vi "Line Linear Fit.vi"(8 "error in":errorcluster, 9 "Keys":refnum<class "1D Array u32.lvclass">, 10 "Y":refnum<class "1D Array f32.lvclass">, 11 "X":refnum<class "1D Array f32.lvclass">) -> (0 "error out":errorcluster, 1 "Keys":refnum<class "1D Array u32.lvclass">, 2 "Offset":refnum<class "1D Array f32.lvclass">, 3 "Slope":refnum<class "1D Array f32.lvclass">)   [LabVIEW 2024, in "G2CPU Line Profile.lvlib"]
uses:
  G2CPU Line Profile.lvlib
  <vilib>/Natan Biesmans/G2CPU GPU and CPU HPC Toolkit/G2CPU Libraries/Arrays/1DArray/f32/1D Array f32.lvclass
  C:/Program Files/National Instruments/LabVIEW 2025/vi.lib/Natan Biesmans/G2CPU GPU and CPU HPC Toolkit/G2CPU Libraries/Arrays/Array/Array Prototype.lvclass
  C:/Program Files/National Instruments/LabVIEW 2025/vi.lib/Natan Biesmans/G2CPU GPU and CPU HPC Toolkit/G2CPU Libraries/Arrays/1DArray/1D Array Prototype.lvclass
  <vilib>/Natan Biesmans/G2CPU GPU and CPU HPC Toolkit/G2CPU Libraries/Arrays/1DArray/u32/1D Array u32.lvclass
  168ab924-3f3a-4db2-9cdf-e3d1f64b3aa0.vi
  0e2f45cd-41b9-45c1-a9b9-d013222e4af8.vi
  1f0995f6-d0b0-43f5-a6c2-40305d76432c.vi
  3dc9b0e7-5c3c-4335-af04-05c96a1d9579.vi
  eb82d686-69ce-41bb-8ade-32c9401aa96d.vi
  546f2740-fcf4-4d92-a73d-2c7a874bd7f8.vi
  a3d83607-c738-4256-a254-dc9f631af114.vi
  ee062472-8682-463b-83ff-a41c4e45bcd6.vi
  10035bee-21f0-4aab-9f26-4981b32c8c4e.vi
  73cb6350-5534-4d8a-b705-d1efc928d9b2.vi
  14413830-6ba5-421c-b5be-a333aee7ddc9.vi
  661186f9-425e-4888-8acc-81e64f3364c9.vi
  700b6014-a647-433f-a561-5befaa5067fc.vi
  6550b275-f30d-4b92-a02f-5e7bb5c687a5.vi
  820307c5-4fb2-499f-9659-8297cac63ad2.vi
  c3e4c011-86fb-4641-86fe-1625446fe100.vi
  84420d7e-1cd2-4cf3-975b-0a4a3f4d0c7e.vi
  168ab924-3f3a-4db2-9cdf-e3d1f64b3aa0.vi/6e6c067d-5978-424b-80f1-88c3a0ffd5ec.vi
  168ab924-3f3a-4db2-9cdf-e3d1f64b3aa0.vi/102d6add-a795-4112-b477-17e7a72fc443.vi
  168ab924-3f3a-4db2-9cdf-e3d1f64b3aa0.vi/cd277467-b234-4cce-8fd2-a3bd8d6792e1.vi
  0e2f45cd-41b9-45c1-a9b9-d013222e4af8.vi/6197f869-f6d4-49b3-9b2c-cc979b422c2e.vi
  0e2f45cd-41b9-45c1-a9b9-d013222e4af8.vi/a7e86dbb-b4c0-485c-89c5-522e60ee265c.vi
  1f0995f6-d0b0-43f5-a6c2-40305d76432c.vi/d0fc544b-4239-492d-8a0f-f99369e9c7ae.vi
  1f0995f6-d0b0-43f5-a6c2-40305d76432c.vi/3d9e75e3-2a93-4e4c-a851-83639de319bb.vi
  3dc9b0e7-5c3c-4335-af04-05c96a1d9579.vi/c9dded55-ca8d-4e9c-82fa-de3705eb1997.vi
  3dc9b0e7-5c3c-4335-af04-05c96a1d9579.vi/77657c34-d6a5-4eb3-ad2b-a32f9da8910d.vi
  eb82d686-69ce-41bb-8ade-32c9401aa96d.vi/6197f869-f6d4-49b3-9b2c-cc979b422c2e.vi
  eb82d686-69ce-41bb-8ade-32c9401aa96d.vi/a7e86dbb-b4c0-485c-89c5-522e60ee265c.vi
  546f2740-fcf4-4d92-a73d-2c7a874bd7f8.vi/c9dded55-ca8d-4e9c-82fa-de3705eb1997.vi
  546f2740-fcf4-4d92-a73d-2c7a874bd7f8.vi/77657c34-d6a5-4eb3-ad2b-a32f9da8910d.vi
  a3d83607-c738-4256-a254-dc9f631af114.vi/c9dded55-ca8d-4e9c-82fa-de3705eb1997.vi
  a3d83607-c738-4256-a254-dc9f631af114.vi/77657c34-d6a5-4eb3-ad2b-a32f9da8910d.vi
  ee062472-8682-463b-83ff-a41c4e45bcd6.vi/6197f869-f6d4-49b3-9b2c-cc979b422c2e.vi
  ee062472-8682-463b-83ff-a41c4e45bcd6.vi/a7e86dbb-b4c0-485c-89c5-522e60ee265c.vi
  10035bee-21f0-4aab-9f26-4981b32c8c4e.vi/c9dded55-ca8d-4e9c-82fa-de3705eb1997.vi
  10035bee-21f0-4aab-9f26-4981b32c8c4e.vi/77657c34-d6a5-4eb3-ad2b-a32f9da8910d.vi
  73cb6350-5534-4d8a-b705-d1efc928d9b2.vi/6197f869-f6d4-49b3-9b2c-cc979b422c2e.vi
  73cb6350-5534-4d8a-b705-d1efc928d9b2.vi/a7e86dbb-b4c0-485c-89c5-522e60ee265c.vi
  14413830-6ba5-421c-b5be-a333aee7ddc9.vi/1bf6e03b-eb75-45f6-9764-49dc38a3a024.vi
  14413830-6ba5-421c-b5be-a333aee7ddc9.vi/2da4419f-02df-47a7-be00-1b7e0871fa33.vi
  661186f9-425e-4888-8acc-81e64f3364c9.vi/d0fc544b-4239-492d-8a0f-f99369e9c7ae.vi
  661186f9-425e-4888-8acc-81e64f3364c9.vi/3d9e75e3-2a93-4e4c-a851-83639de319bb.vi
  700b6014-a647-433f-a561-5befaa5067fc.vi/1bf6e03b-eb75-45f6-9764-49dc38a3a024.vi
  700b6014-a647-433f-a561-5befaa5067fc.vi/2da4419f-02df-47a7-be00-1b7e0871fa33.vi
  6550b275-f30d-4b92-a02f-5e7bb5c687a5.vi/46771f49-eb1d-473b-8e81-f516cef50a4e.vi
  6550b275-f30d-4b92-a02f-5e7bb5c687a5.vi/dc76f8e4-64fa-456a-8549-7a4b6936c4c9.vi
  6550b275-f30d-4b92-a02f-5e7bb5c687a5.vi/7e60ddfb-e748-4c0c-85da-e395a1b7978d.vi
  6550b275-f30d-4b92-a02f-5e7bb5c687a5.vi/d2eceff7-f641-4ce4-acfa-e9e293a3c877.vi
  6550b275-f30d-4b92-a02f-5e7bb5c687a5.vi/b737122b-4036-448b-abd3-e2701355e828.vi
  820307c5-4fb2-499f-9659-8297cac63ad2.vi/6197f869-f6d4-49b3-9b2c-cc979b422c2e.vi
  820307c5-4fb2-499f-9659-8297cac63ad2.vi/a7e86dbb-b4c0-485c-89c5-522e60ee265c.vi
  c3e4c011-86fb-4641-86fe-1625446fe100.vi/1bf6e03b-eb75-45f6-9764-49dc38a3a024.vi
  c3e4c011-86fb-4641-86fe-1625446fe100.vi/2da4419f-02df-47a7-be00-1b7e0871fa33.vi
  84420d7e-1cd2-4cf3-975b-0a4a3f4d0c7e.vi/46771f49-eb1d-473b-8e81-f516cef50a4e.vi
  84420d7e-1cd2-4cf3-975b-0a4a3f4d0c7e.vi/dc76f8e4-64fa-456a-8549-7a4b6936c4c9.vi
  84420d7e-1cd2-4cf3-975b-0a4a3f4d0c7e.vi/7e60ddfb-e748-4c0c-85da-e395a1b7978d.vi
  84420d7e-1cd2-4cf3-975b-0a4a3f4d0c7e.vi/d2eceff7-f641-4ce4-acfa-e9e293a3c877.vi
  84420d7e-1cd2-4cf3-975b-0a4a3f4d0c7e.vi/b737122b-4036-448b-abd3-e2701355e828.vi
  0e2f45cd-41b9-45c1-a9b9-d013222e4af8.vi/6197f869-f6d4-49b3-9b2c-cc979b422c2e.vi/3e802c67-fb96-46a3-ae13-4994a8508b4f.vi
  0e2f45cd-41b9-45c1-a9b9-d013222e4af8.vi/6197f869-f6d4-49b3-9b2c-cc979b422c2e.vi/5a50fc67-79e7-4972-80c2-92243cd53dd4.vi
  0e2f45cd-41b9-45c1-a9b9-d013222e4af8.vi/a7e86dbb-b4c0-485c-89c5-522e60ee265c.vi/730f6c57-5c0b-4ee9-b61e-75067b25222b.vi
  0e2f45cd-41b9-45c1-a9b9-d013222e4af8.vi/a7e86dbb-b4c0-485c-89c5-522e60ee265c.vi/096b8799-7810-404e-baca-ba9279cec4bd.vi
  0e2f45cd-41b9-45c1-a9b9-d013222e4af8.vi/a7e86dbb-b4c0-485c-89c5-522e60ee265c.vi/0f1a5a47-bcc5-4796-ac31-8dfcfbc0d7d1.vi
  0e2f45cd-41b9-45c1-a9b9-d013222e4af8.vi/a7e86dbb-b4c0-485c-89c5-522e60ee265c.vi/89f12e17-3330-4b72-ad8f-8dd636660732.vi
  1f0995f6-d0b0-43f5-a6c2-40305d76432c.vi/d0fc544b-4239-492d-8a0f-f99369e9c7ae.vi/3587aa3f-97a0-4074-a424-c31da557ec96.vi
  1f0995f6-d0b0-43f5-a6c2-40305d76432c.vi/d0fc544b-4239-492d-8a0f-f99369e9c7ae.vi/6058dca8-195d-4566-b47b-6d6a1c5af61f.vi
  1f0995f6-d0b0-43f5-a6c2-40305d76432c.vi/3d9e75e3-2a93-4e4c-a851-83639de319bb.vi/730f6c57-5c0b-4ee9-b61e-75067b25222b.vi
  1f0995f6-d0b0-43f5-a6c2-40305d76432c.vi/3d9e75e3-2a93-4e4c-a851-83639de319bb.vi/096b8799-7810-404e-baca-ba9279cec4bd.vi
  1f0995f6-d0b0-43f5-a6c2-40305d76432c.vi/3d9e75e3-2a93-4e4c-a851-83639de319bb.vi/0f1a5a47-bcc5-4796-ac31-8dfcfbc0d7d1.vi
  1f0995f6-d0b0-43f5-a6c2-40305d76432c.vi/3d9e75e3-2a93-4e4c-a851-83639de319bb.vi/89f12e17-3330-4b72-ad8f-8dd636660732.vi
  eb82d686-69ce-41bb-8ade-32c9401aa96d.vi/6197f869-f6d4-49b3-9b2c-cc979b422c2e.vi/3e802c67-fb96-46a3-ae13-4994a8508b4f.vi
  eb82d686-69ce-41bb-8ade-32c9401aa96d.vi/6197f869-f6d4-49b3-9b2c-cc979b422c2e.vi/5a50fc67-79e7-4972-80c2-92243cd53dd4.vi
  eb82d686-69ce-41bb-8ade-32c9401aa96d.vi/a7e86dbb-b4c0-485c-89c5-522e60ee265c.vi/730f6c57-5c0b-4ee9-b61e-75067b25222b.vi
  eb82d686-69ce-41bb-8ade-32c9401aa96d.vi/a7e86dbb-b4c0-485c-89c5-522e60ee265c.vi/096b8799-7810-404e-baca-ba9279cec4bd.vi
  eb82d686-69ce-41bb-8ade-32c9401aa96d.vi/a7e86dbb-b4c0-485c-89c5-522e60ee265c.vi/0f1a5a47-bcc5-4796-ac31-8dfcfbc0d7d1.vi
  eb82d686-69ce-41bb-8ade-32c9401aa96d.vi/a7e86dbb-b4c0-485c-89c5-522e60ee265c.vi/89f12e17-3330-4b72-ad8f-8dd636660732.vi
  ee062472-8682-463b-83ff-a41c4e45bcd6.vi/6197f869-f6d4-49b3-9b2c-cc979b422c2e.vi/3e802c67-fb96-46a3-ae13-4994a8508b4f.vi
  ee062472-8682-463b-83ff-a41c4e45bcd6.vi/6197f869-f6d4-49b3-9b2c-cc979b422c2e.vi/5a50fc67-79e7-4972-80c2-92243cd53dd4.vi
  ee062472-8682-463b-83ff-a41c4e45bcd6.vi/a7e86dbb-b4c0-485c-89c5-522e60ee265c.vi/730f6c57-5c0b-4ee9-b61e-75067b25222b.vi
  ee062472-8682-463b-83ff-a41c4e45bcd6.vi/a7e86dbb-b4c0-485c-89c5-522e60ee265c.vi/096b8799-7810-404e-baca-ba9279cec4bd.vi
  ee062472-8682-463b-83ff-a41c4e45bcd6.vi/a7e86dbb-b4c0-485c-89c5-522e60ee265c.vi/0f1a5a47-bcc5-4796-ac31-8dfcfbc0d7d1.vi
  ee062472-8682-463b-83ff-a41c4e45bcd6.vi/a7e86dbb-b4c0-485c-89c5-522e60ee265c.vi/89f12e17-3330-4b72-ad8f-8dd636660732.vi
  73cb6350-5534-4d8a-b705-d1efc928d9b2.vi/6197f869-f6d4-49b3-9b2c-cc979b422c2e.vi/3e802c67-fb96-46a3-ae13-4994a8508b4f.vi
  73cb6350-5534-4d8a-b705-d1efc928d9b2.vi/6197f869-f6d4-49b3-9b2c-cc979b422c2e.vi/5a50fc67-79e7-4972-80c2-92243cd53dd4.vi
  73cb6350-5534-4d8a-b705-d1efc928d9b2.vi/a7e86dbb-b4c0-485c-89c5-522e60ee265c.vi/730f6c57-5c0b-4ee9-b61e-75067b25222b.vi
  73cb6350-5534-4d8a-b705-d1efc928d9b2.vi/a7e86dbb-b4c0-485c-89c5-522e60ee265c.vi/096b8799-7810-404e-baca-ba9279cec4bd.vi
  73cb6350-5534-4d8a-b705-d1efc928d9b2.vi/a7e86dbb-b4c0-485c-89c5-522e60ee265c.vi/0f1a5a47-bcc5-4796-ac31-8dfcfbc0d7d1.vi
  73cb6350-5534-4d8a-b705-d1efc928d9b2.vi/a7e86dbb-b4c0-485c-89c5-522e60ee265c.vi/89f12e17-3330-4b72-ad8f-8dd636660732.vi
  14413830-6ba5-421c-b5be-a333aee7ddc9.vi/1bf6e03b-eb75-45f6-9764-49dc38a3a024.vi/3e802c67-fb96-46a3-ae13-4994a8508b4f.vi
  14413830-6ba5-421c-b5be-a333aee7ddc9.vi/1bf6e03b-eb75-45f6-9764-49dc38a3a024.vi/5a50fc67-79e7-4972-80c2-92243cd53dd4.vi
  14413830-6ba5-421c-b5be-a333aee7ddc9.vi/2da4419f-02df-47a7-be00-1b7e0871fa33.vi/730f6c57-5c0b-4ee9-b61e-75067b25222b.vi
  14413830-6ba5-421c-b5be-a333aee7ddc9.vi/2da4419f-02df-47a7-be00-1b7e0871fa33.vi/096b8799-7810-404e-baca-ba9279cec4bd.vi
  14413830-6ba5-421c-b5be-a333aee7ddc9.vi/2da4419f-02df-47a7-be00-1b7e0871fa33.vi/0f1a5a47-bcc5-4796-ac31-8dfcfbc0d7d1.vi
  14413830-6ba5-421c-b5be-a333aee7ddc9.vi/2da4419f-02df-47a7-be00-1b7e0871fa33.vi/89f12e17-3330-4b72-ad8f-8dd636660732.vi
  661186f9-425e-4888-8acc-81e64f3364c9.vi/d0fc544b-4239-492d-8a0f-f99369e9c7ae.vi/3587aa3f-97a0-4074-a424-c31da557ec96.vi
  661186f9-425e-4888-8acc-81e64f3364c9.vi/d0fc544b-4239-492d-8a0f-f99369e9c7ae.vi/6058dca8-195d-4566-b47b-6d6a1c5af61f.vi
  661186f9-425e-4888-8acc-81e64f3364c9.vi/3d9e75e3-2a93-4e4c-a851-83639de319bb.vi/730f6c57-5c0b-4ee9-b61e-75067b25222b.vi
  661186f9-425e-4888-8acc-81e64f3364c9.vi/3d9e75e3-2a93-4e4c-a851-83639de319bb.vi/096b8799-7810-404e-baca-ba9279cec4bd.vi
  661186f9-425e-4888-8acc-81e64f3364c9.vi/3d9e75e3-2a93-4e4c-a851-83639de319bb.vi/0f1a5a47-bcc5-4796-ac31-8dfcfbc0d7d1.vi
  661186f9-425e-4888-8acc-81e64f3364c9.vi/3d9e75e3-2a93-4e4c-a851-83639de319bb.vi/89f12e17-3330-4b72-ad8f-8dd636660732.vi
  700b6014-a647-433f-a561-5befaa5067fc.vi/1bf6e03b-eb75-45f6-9764-49dc38a3a024.vi/3e802c67-fb96-46a3-ae13-4994a8508b4f.vi
  700b6014-a647-433f-a561-5befaa5067fc.vi/1bf6e03b-eb75-45f6-9764-49dc38a3a024.vi/5a50fc67-79e7-4972-80c2-92243cd53dd4.vi
  700b6014-a647-433f-a561-5befaa5067fc.vi/2da4419f-02df-47a7-be00-1b7e0871fa33.vi/730f6c57-5c0b-4ee9-b61e-75067b25222b.vi
  700b6014-a647-433f-a561-5befaa5067fc.vi/2da4419f-02df-47a7-be00-1b7e0871fa33.vi/096b8799-7810-404e-baca-ba9279cec4bd.vi
  700b6014-a647-433f-a561-5befaa5067fc.vi/2da4419f-02df-47a7-be00-1b7e0871fa33.vi/0f1a5a47-bcc5-4796-ac31-8dfcfbc0d7d1.vi
  700b6014-a647-433f-a561-5befaa5067fc.vi/2da4419f-02df-47a7-be00-1b7e0871fa33.vi/89f12e17-3330-4b72-ad8f-8dd636660732.vi
  6550b275-f30d-4b92-a02f-5e7bb5c687a5.vi/dc76f8e4-64fa-456a-8549-7a4b6936c4c9.vi/3e802c67-fb96-46a3-ae13-4994a8508b4f.vi
  6550b275-f30d-4b92-a02f-5e7bb5c687a5.vi/dc76f8e4-64fa-456a-8549-7a4b6936c4c9.vi/5a50fc67-79e7-4972-80c2-92243cd53dd4.vi
  820307c5-4fb2-499f-9659-8297cac63ad2.vi/6197f869-f6d4-49b3-9b2c-cc979b422c2e.vi/3e802c67-fb96-46a3-ae13-4994a8508b4f.vi
  820307c5-4fb2-499f-9659-8297cac63ad2.vi/6197f869-f6d4-49b3-9b2c-cc979b422c2e.vi/5a50fc67-79e7-4972-80c2-92243cd53dd4.vi
  820307c5-4fb2-499f-9659-8297cac63ad2.vi/a7e86dbb-b4c0-485c-89c5-522e60ee265c.vi/730f6c57-5c0b-4ee9-b61e-75067b25222b.vi
  820307c5-4fb2-499f-9659-8297cac63ad2.vi/a7e86dbb-b4c0-485c-89c5-522e60ee265c.vi/096b8799-7810-404e-baca-ba9279cec4bd.vi
  820307c5-4fb2-499f-9659-8297cac63ad2.vi/a7e86dbb-b4c0-485c-89c5-522e60ee265c.vi/0f1a5a47-bcc5-4796-ac31-8dfcfbc0d7d1.vi
  820307c5-4fb2-499f-9659-8297cac63ad2.vi/a7e86dbb-b4c0-485c-89c5-522e60ee265c.vi/89f12e17-3330-4b72-ad8f-8dd636660732.vi
  c3e4c011-86fb-4641-86fe-1625446fe100.vi/1bf6e03b-eb75-45f6-9764-49dc38a3a024.vi/3e802c67-fb96-46a3-ae13-4994a8508b4f.vi
  c3e4c011-86fb-4641-86fe-1625446fe100.vi/1bf6e03b-eb75-45f6-9764-49dc38a3a024.vi/5a50fc67-79e7-4972-80c2-92243cd53dd4.vi
  c3e4c011-86fb-4641-86fe-1625446fe100.vi/2da4419f-02df-47a7-be00-1b7e0871fa33.vi/730f6c57-5c0b-4ee9-b61e-75067b25222b.vi
  c3e4c011-86fb-4641-86fe-1625446fe100.vi/2da4419f-02df-47a7-be00-1b7e0871fa33.vi/096b8799-7810-404e-baca-ba9279cec4bd.vi
  c3e4c011-86fb-4641-86fe-1625446fe100.vi/2da4419f-02df-47a7-be00-1b7e0871fa33.vi/0f1a5a47-bcc5-4796-ac31-8dfcfbc0d7d1.vi
  c3e4c011-86fb-4641-86fe-1625446fe100.vi/2da4419f-02df-47a7-be00-1b7e0871fa33.vi/89f12e17-3330-4b72-ad8f-8dd636660732.vi
  84420d7e-1cd2-4cf3-975b-0a4a3f4d0c7e.vi/dc76f8e4-64fa-456a-8549-7a4b6936c4c9.vi/3e802c67-fb96-46a3-ae13-4994a8508b4f.vi
  84420d7e-1cd2-4cf3-975b-0a4a3f4d0c7e.vi/dc76f8e4-64fa-456a-8549-7a4b6936c4c9.vi/5a50fc67-79e7-4972-80c2-92243cd53dd4.vi
  1f0995f6-d0b0-43f5-a6c2-40305d76432c.vi/d0fc544b-4239-492d-8a0f-f99369e9c7ae.vi/6058dca8-195d-4566-b47b-6d6a1c5af61f.vi/77c7badc-ed81-4514-99c1-20d37f4e5ecc.vi
  1f0995f6-d0b0-43f5-a6c2-40305d76432c.vi/d0fc544b-4239-492d-8a0f-f99369e9c7ae.vi/6058dca8-195d-4566-b47b-6d6a1c5af61f.vi/eb76fa01-6782-47b4-b34f-9eb474c9cc78.vi
  661186f9-425e-4888-8acc-81e64f3364c9.vi/d0fc544b-4239-492d-8a0f-f99369e9c7ae.vi/6058dca8-195d-4566-b47b-6d6a1c5af61f.vi/77c7badc-ed81-4514-99c1-20d37f4e5ecc.vi
  661186f9-425e-4888-8acc-81e64f3364c9.vi/d0fc544b-4239-492d-8a0f-f99369e9c7ae.vi/6058dca8-195d-4566-b47b-6d6a1c5af61f.vi/eb76fa01-6782-47b4-b34f-9eb474c9cc78.vi
  <vilib>/Natan Biesmans/G2CPU GPU and CPU HPC Toolkit/G2CPU Libraries/Arrays/1DArray/1D Array Prototype.lvclass
  <vilib>/Natan Biesmans/G2CPU GPU and CPU HPC Toolkit/G2CPU Libraries/Arrays/SubVI/Lock Arrays.vi
  <vilib>/Natan Biesmans/G2CPU GPU and CPU HPC Toolkit/G2CPU Libraries/Arrays/Array/G2CPU Get Array Pointer.vi
  <vilib>/Natan Biesmans/G2CPU GPU and CPU HPC Toolkit/ArrayFire Driver/VIs/count by key.vi
  <vilib>/Natan Biesmans/G2CPU GPU and CPU HPC Toolkit/G2CPU Libraries/Arrays/Array/G2CPU Unlock Array.vi
  <vilib>/Natan Biesmans/G2CPU GPU and CPU HPC Toolkit/G2CPU Libraries/Arrays/Array/G2CPU Set Array Pointer.vi
  <vilib>/Natan Biesmans/G2CPU GPU and CPU HPC Toolkit/ArrayFire Driver/VIs/Run as Multi Device.vi
  <vilib>/Natan Biesmans/G2CPU GPU and CPU HPC Toolkit/ArrayFire Driver/VIs/iszero.vi
  <vilib>/Natan Biesmans/G2CPU GPU and CPU HPC Toolkit/ArrayFire Driver/VIs/sub.vi
  <vilib>/Natan Biesmans/G2CPU GPU and CPU HPC Toolkit/ArrayFire Driver/VIs/release array.vi
  <vilib>/Natan Biesmans/G2CPU GPU and CPU HPC Toolkit/G2CPU Libraries/Manage Environment/Find AF DLL.vi
  <vilib>/Natan Biesmans/G2CPU GPU and CPU HPC Toolkit/ArrayFire Driver/subvi/Error Converter (ErrCode or Status).vi
  <vilib>/Natan Biesmans/G2CPU GPU and CPU HPC Toolkit/ArrayFire Driver/VIs/cast.vi
  <vilib>/Natan Biesmans/G2CPU GPU and CPU HPC Toolkit/ArrayFire Driver/VIs/add.vi
  <vilib>/Natan Biesmans/G2CPU GPU and CPU HPC Toolkit/G2CPU Libraries/Arrays/SubVI/is 1D.vi
  <vilib>/Natan Biesmans/G2CPU GPU and CPU HPC Toolkit/ArrayFire Driver/VIs/pow.vi
  <vilib>/Natan Biesmans/G2CPU GPU and CPU HPC Toolkit/ArrayFire Driver/VIs/mul.vi
  <vilib>/Natan Biesmans/G2CPU GPU and CPU HPC Toolkit/ArrayFire Driver/VIs/sum by key.vi
  <vilib>/Natan Biesmans/G2CPU GPU and CPU HPC Toolkit/ArrayFire Driver/VIs/div.vi
  <vilib>/Natan Biesmans/G2CPU GPU and CPU HPC Toolkit/G2CPU Libraries/Arrays/Array/Array Prototype.lvclass
  <vilib>/Natan Biesmans/G2CPU GPU and CPU HPC Toolkit/G2CPU Libraries/Arrays/DataTypes/f32/f32.lvclass
  <vilib>/Natan Biesmans/G2CPU GPU and CPU HPC Toolkit/G2CPU Libraries/Arrays/DataTypes/U32/U32.lvclass
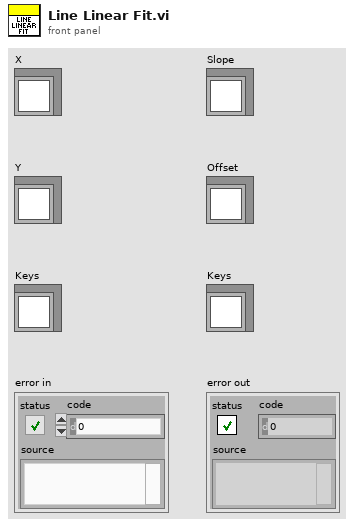
[diagram p1: front panel]
types:
  T1 = typedef "AF.lvlib/Dim4.ctl" = cluster{"Dim 0":u64, "Dim 1":u64, "Dim 2":u64, "Dim 3":u64}
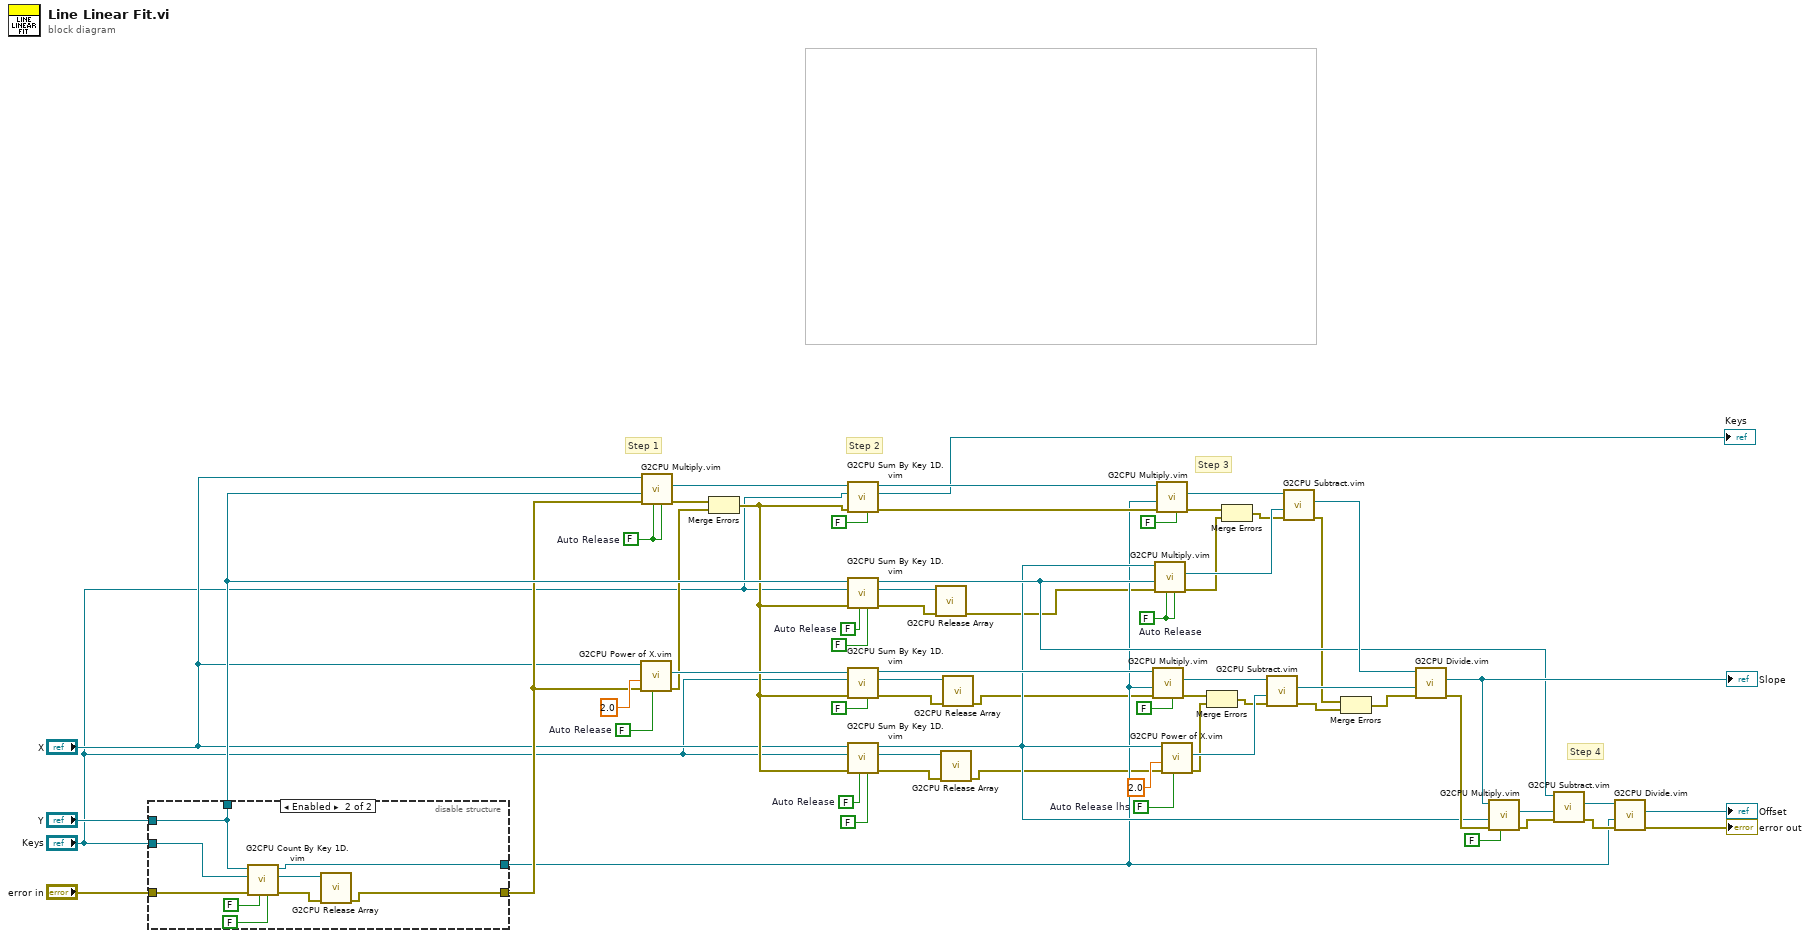
[diagram p0: block diagram]
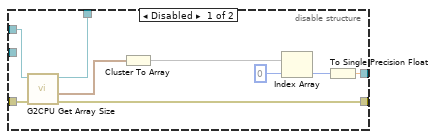
[diagram p2: hidden frame]
diagram:
  w20 = FALSE  # Auto Release
  w21 = FALSE  # Auto Release
  w41 = FALSE  # Auto Release lhs
  w42 = FALSE  # Auto Release
  w47 = FALSE  # Auto Release
  w48 = FALSE  # Auto Release
  # "Step 4"
  # "Step 3"
  # "Step 2"
  # "Step 1"
  n1 = disable-structure shown="Enabled" {
    disable-tunnel: [w73 w83] -> w49
    disable-tunnel: [w70 w75] -> w26
    disable-tunnel: "error in" -> [w69 w82]
    disable-tunnel: [w68 w78] -> w24
    disable-tunnel: "Y" -> [w67 w83]
    disable-tunnel: "Keys" -> [_ w80]
    frame Disabled {
      n2 = call <vilib>:"G2CPU Get Array Size.vi"("error in (no error)"=w69, "Array in"=w67) -> ("error out"=w70:errorcluster, "Array Size"=w74:T1, "Array out"=w73:refnum<class "1D Array f32.lvclass">)  [unwired: 6 in, 1 out]
      n3 = Cluster To Array(cluster=w74) -> (array=w72:u64[])
      n4 = Index Array(array=w72, index=0 ("Dim")) -> (element=w71:u64)
      n5 = To Single Precision Float(number=w71) -> (single precision float=w68:sgl)
    }
    frame Enabled {
      n6 = call "G2CPU Count By Key 1D.vim"("Auto Release Keys (Enabled)"=FALSE, "Auto Release Array In (Enabled)"=FALSE ("Auto Release (Enabled)"), "error in (no error)"=w82, "Array Keys 1D U32"=w80, "Array First"=w83) -> ("error out"=w77:errorcluster, "Array Keys"=w76:refnum<class "1D Array u32.lvclass">, "Array out"=w78:refnum<class "1D Array u32.lvclass">)  [unwired: 4 in]
      n7 = call <vilib>:"G2CPU Release Array.vi"("error in (no error)"=w77, "Array in"=w76) -> ("error out"=w75:errorcluster)  [unwired: 9 in]
    }
  }
  n8 = call "G2CPU Power of X.vim"("Auto Release lhs (Enabled)"=w47, "error in (no error)"=w26, "Array rhs"=sgl 2.0 ("val"), "Array lhs"="X") -> ("error out"=w45:errorcluster, "Array Result"=w64:refnum<class "1D Array f32.lvclass">)  [unwired: 6 in]
  n9 = call "G2CPU Multiply.vim"("Auto Release rhs"=w48, "Auto Release lhs"=w48, "error in (no error)"=w26, "Array rhs"=w49, "Array lhs"="X") -> ("error out"=w46:errorcluster, "Array Result"=w63:refnum<class "1D Array f32.lvclass">)  [unwired: 5 in]
  n10 = Merge Errors(w46, w45) -> (w44:errorcluster)
  n11 = call "G2CPU Sum By Key 1D.vim"("Auto Release Keys (Enabled)"=FALSE, "error in (no error)"=w44, "Array Key 1D U32"="Keys", "Array In"=w63) -> ("error out"=w43:errorcluster, "Array Keys"=→"Keys":refnum<class "1D Array u32.lvclass">, "Array Out"=w61:refnum<class "1D Array f32.lvclass">)  [unwired: 5 in]
  n12 = call "G2CPU Sum By Key 1D.vim"("Auto Release Keys (Enabled)"=FALSE, "Auto Release Array In (Enabled)"=w20, "error in (no error)"=w44, "Array Key 1D U32"="Keys", "Array In"=w49) -> ("error out"=w5:errorcluster, "Array Keys"=w12:refnum<class "1D Array u32.lvclass">, "Array Out"=w52:refnum<class "1D Array f32.lvclass">)  [unwired: 4 in]
  n13 = call "G2CPU Sum By Key 1D.vim"("Auto Release Keys (Enabled)"=FALSE, "error in (no error)"=w44, "Array Key 1D U32"="Keys", "Array In"=w64) -> ("error out"=w7:errorcluster, "Array Keys"=w11:refnum<class "1D Array u32.lvclass">, "Array Out"=w62:refnum<class "1D Array f32.lvclass">)  [unwired: 5 in]
  n14 = call "G2CPU Sum By Key 1D.vim"("Auto Release Keys (Enabled)"=FALSE, "Auto Release Array In (Enabled)"=w21, "error in (no error)"=w44, "Array Key 1D U32"="Keys", "Array In"="X") -> ("error out"=w9:errorcluster, "Array Keys"=w10:refnum<class "1D Array u32.lvclass">, "Array Out"=w27:refnum<class "1D Array f32.lvclass">)  [unwired: 4 in]
  n15 = call <vilib>:"G2CPU Release Array.vi"("error in (no error)"=w5, "Array in"=w12) -> ("error out"=w4:errorcluster)  [unwired: 9 in]
  n16 = call <vilib>:"G2CPU Release Array.vi"("error in (no error)"=w9, "Array in"=w10) -> ("error out"=w8:errorcluster)  [unwired: 9 in]
  n17 = call <vilib>:"G2CPU Release Array.vi"("error in (no error)"=w7, "Array in"=w11) -> ("error out"=w6:errorcluster)  [unwired: 9 in]
  n18 = call "G2CPU Multiply.vim"("Auto Release rhs"=FALSE, "error in (no error)"=w6, "Array rhs"=w24, "Array lhs"=w62) -> ("error out"=w37:errorcluster, "Array Result"=w57:refnum<class "1D Array f32.lvclass">)  [unwired: 6 in]
  n19 = call "G2CPU Multiply.vim"("Auto Release rhs"=w42, "Auto Release lhs"=w42, "error in (no error)"=w4, "Array rhs"=w52, "Array lhs"=w27) -> ("error out"=w39:errorcluster, "Array Result"=w60:refnum<class "1D Array f32.lvclass">)  [unwired: 5 in]
  n20 = call "G2CPU Multiply.vim"("Auto Release rhs"=FALSE, "error in (no error)"=w43, "Array rhs"=w24, "Array lhs"=w61) -> ("error out"=w40:errorcluster, "Array Result"=w59:refnum<class "1D Array f32.lvclass">)  [unwired: 6 in]
  n21 = call "G2CPU Power of X.vim"("Auto Release lhs (Enabled)"=w41, "error in (no error)"=w8, "Array rhs"=sgl 2.0 ("val"), "Array lhs"=w27) -> ("error out"=w36:errorcluster, "Array Result"=w58:refnum<class "1D Array f32.lvclass">)  [unwired: 6 in]
  n22 = Merge Errors(w37, w36) -> (w35:errorcluster)
  n23 = Merge Errors(w40, w39) -> (w38:errorcluster)
  n24 = call "G2CPU Subtract.vim"("error in (no error)"=w35, "Array rhs"=w58, "Array lhs"=w57) -> ("error out"=w33:errorcluster, "Array Result"=w55:refnum<class "1D Array f32.lvclass">)  [unwired: 7 in]
  n25 = call "G2CPU Subtract.vim"("error in (no error)"=w38, "Array rhs"=w60, "Array lhs"=w59) -> ("error out"=w34:errorcluster, "Array Result"=w54:refnum<class "1D Array f32.lvclass">)  [unwired: 7 in]
  n26 = Merge Errors(w34, w33) -> (w32:errorcluster)
  n27 = call "G2CPU Divide.vim"("error in (no error)"=w32, "Array rhs"=w55, "Array lhs"=w54) -> ("error out"=w31:errorcluster, "Array Result"=w56:refnum<class "1D Array f32.lvclass">)  [unwired: 7 in]
  "Slope" <- w56
  n28 = call "G2CPU Multiply.vim"("Auto Release lhs"=FALSE, "error in (no error)"=w31, "Array rhs"=w27, "Array lhs"=w56) -> ("error out"=w30:errorcluster, "Array Result"=w53:refnum<class "1D Array f32.lvclass">)  [unwired: 6 in]
  n29 = call "G2CPU Subtract.vim"("error in (no error)"=w30, "Array rhs"=w53, "Array lhs"=w52) -> ("error out"=w29:errorcluster, "Array Result"=w51:refnum<class "1D Array f32.lvclass">)  [unwired: 7 in]
  n30 = call "G2CPU Divide.vim"("error in (no error)"=w29, "Array rhs"=w24, "Array lhs"=w51) -> ("error out"=→"error out":errorcluster, "Array Result"=→"Offset":refnum<class "1D Array f32.lvclass">)  [unwired: 7 in]
